vi "test.vi"() -> ()   [LabVIEW 2010]
uses:
  motion_correction_cluster.ctl
panel:
  out "left over":u16[](array[numeric])
  in  "channel":i8
  in  "Array":u16[](array[numeric])
  out "MC array":u16[](array[numeric])
  out "RAPS data":u64[](array[numeric])
  in  "cluster out":T1={"reception"={"square size"=3, "offset"=0, "# squares out"=0, "mc left over"=[], "raps points length"=7, "raps left over"=[]}, "fft"={"reference"=[]}}
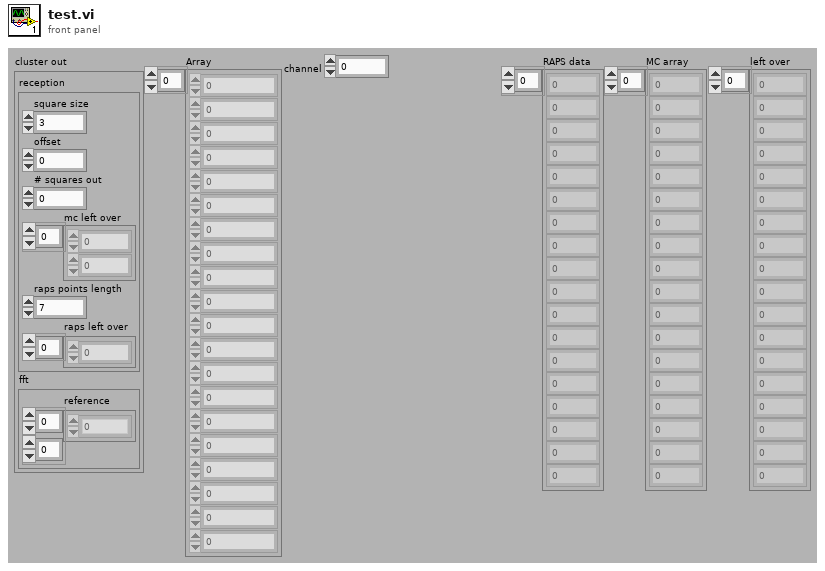
[diagram p1: front panel]
types:
  T1 = typedef "motion_correction_cluster.ctl" = cluster{"reception":cluster{"square size":i32, "offset":i32, "# squares out":i32, "mc left over":u16[], "raps points length":i32, "raps left over":u64[]}, "fft":cluster{"reference":dbl[][]}}
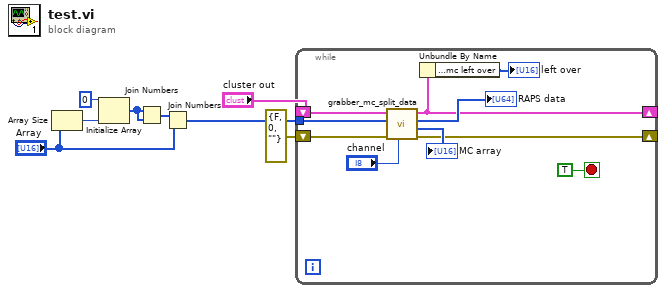
[diagram p0: block diagram]
diagram:
  n1 = Array Size(array="Array") -> (size(s)=w4:i32)
  n2 = Initialize Array(u16 0, w4) -> (w2:u16[])
  n3 = Join Numbers(hi=w2, lo=w2) -> ((hi.lo)=w8:u32[])
  n4 = Join Numbers(hi=w8, lo="Array") -> ((hi.lo)=w7:u64[])
  n5 = while {
    tunnel: w7 -> [w18]
    shift-right: [w10] -> _
    shift-left: "cluster out" -> [w17]
    shift-right: [w13] -> _
    shift-left: errorcluster {"status"=FALSE, "code"=0, "source"=""} ("error out") -> [w16]
    stop <- TRUE stop-if-true
    n6 = call "grabber_mc_split_data.vi"("channel"="channel", "error in (no error)"=w16, "array in"=w18, "cluster in"=w17) -> ("error out"=w13:errorcluster, "MC array"=→"MC array":u16[], "RAPS data"=→"RAPS data":u64[], "cluster out"=w10:T1)  [unwired: 1 in, 3 out]
    n7 = Unbundle By Name(w10) -> ("reception.mc left over"=→"left over":u16[])
  }
